vi "Get CD Item Property Value.vi"(8 "error in (no error)":errorcluster, 10 "CD Item Ref in":T1 format="%.0x", 11 "File Path Parameter in":refnum<class "File Path Parameter.lvclass">) -> (0 "error out":errorcluster, 3 "File Path Parameter out":refnum<class "File Path Parameter.lvclass">)   [LabVIEW 2019, in "CD Parameter Manager API.lvlib" / "File Path Parameter.lvclass"]
uses:
  File Path Parameter.lvclass
  C:/Repositories/CSD_Custom_Device/CSD_Custom_Device/Source/Libraries/CD Parameter Manager API/Parameter Class/Parameter.lvclass
  <vilib>/NI VeriStand/Custom Device API/Custom Device Item Ref.ctl
  Parameter Class/Parameter.lvclass/Parameter.ctl
  File Path Parameter.lvclass/File Path Parameter.ctl
  Parameter Class/Member Accessors/Read Control label.vi
  Member Accessors/Read Value.vi
  Member Accessors/Write Value.vi
  <vilib>/NI VeriStand/Custom Device API/Get Item Property (Path).vi
  <vilib>/NI VeriStand/Custom Device API/Custom Device API.lvlib
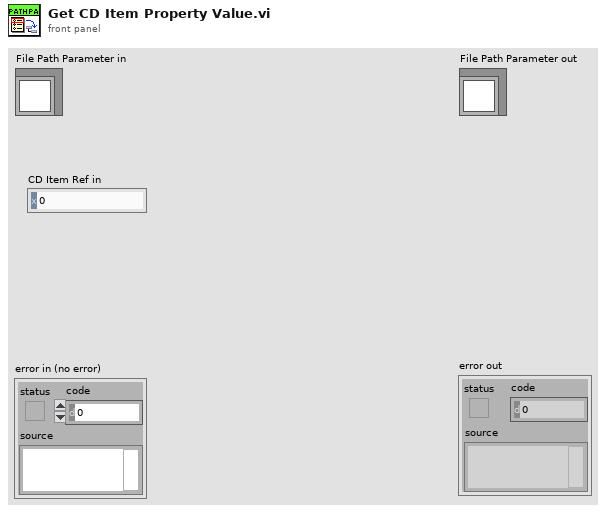
[diagram p1: front panel]
types:
  T1 = typedef "Custom Device API.lvlib/Custom Device Item Ref.ctl" = u64
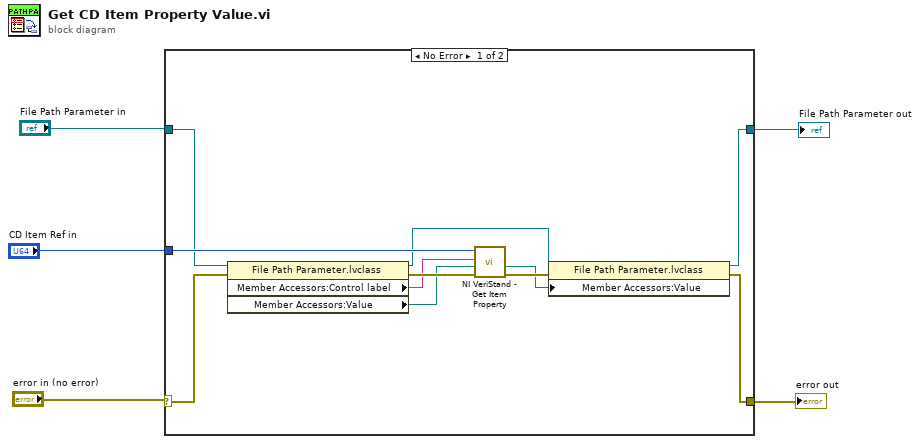
[diagram p0: block diagram]
diagram:
  n1 = case shown="No Error" "error in (no error)" {
    selector: "error in (no error)" -> [w15 w17]
    tunnel: [w9 w17] -> w4
    tunnel: "CD Item Ref in" -> [w16 _]
    tunnel: [w6 w18] -> w5
    tunnel: "File Path Parameter in" -> [w14 w18]
    frame No Error {
      n2 = property class="File Path Parameter.lvclass"(reference=w14, error in=w15) -> (reference out=w7:refnum<class "File Path Parameter.lvclass">, error out=w13:errorcluster, "Member Accessors:Control label"=w12:string, "Member Accessors:Value"=w11:path)
      n3 = call-poly <vilib>:"NI VeriStand - Get Item Property.vi"("error in (no error)"=w13, "Default Value"=w11, "Property Name"=w12, "Item Ref in"=w16) -> ("error out"=w10:errorcluster, "Value"=w8:path)  [unwired: 4 in, 2 out]
      n4 = property class="File Path Parameter.lvclass"(reference=w7, error in=w10, "Member Accessors:Value"=w8) -> (reference out=w6:refnum<class "File Path Parameter.lvclass">, error out=w9:errorcluster)
    }
    frame Error {
    }
  }
  "error out" <- w4
  "File Path Parameter out" <- w5
